vi "FormCalibra3.vi"() -> ()   [LabVIEW 2014]
uses:
  testMachine.ctl
  mainMachine.ctl
  <vilib>/Analysis/baseanly.llb/Mean (DBL).vi
  <vilib>/express/express shared/transition.llb/Dynamic To Waveform Array.vi
  <vilib>/express/express signal manip/GetorSetDDTAttributes/Set DDT Attributes/SetT0.vi
  <vilib>/express/express shared/transition.llb/Waveform Array To Dynamic.vi
  <vilib>/express/express signal manip/GetorSetDDTAttributes/Set DDT Attributes/Set DDT Properties.xnode
  <vilib>/Analysis/NI_AALBase.lvlib
panel:
  in  "buttonAcquisition":bool
  in  "editSetWaitTime":u32 caption="Tempo entre ciclos (ms)" max=999 step=1 format="%0d"
  in  "stop":bool
  out "ledSpeed":bool caption="Velocidade"
  out "error out":errorcluster
  out "ledAcquireState":bool caption="Acquire State"
  out "editTotalLowerLimit":dbl
  out "editCountLowerLimit":dbl
  out "editTotalUpperLimit":dbl
  out "editCountUpperLimit":dbl
  out "ledEnsaio 3":bool
  out "ledBrakeState":bool caption="Brake State"
  out "ledExitState":bool caption="Exit State"
  out "ledMotorState":bool caption="Motor State"
  out "ledInit2State":bool caption="Init State"
  out "ledBlockState":bool caption="Block State"
  out "ledRunningState":bool caption="Running State"
  out "ledReadyState":bool caption="Ready State"
  out "ledInitState":bool caption="Init State"
  out "mainMachine":T1
  out "testMachine":T2=enum."finish"
  in  "editSetPathToFile":path
  out "ledForce":bool caption="Célula de Carga"
  out "ledEngSpeed":bool caption="Rotação"
  out "ledTempB":bool caption="Temperatura B"
  out "ledTempA":bool caption="Temperatura A"
  out "ledTempRef":bool caption="Tempertura (Ref)"
  in  "buttonStop":bool
  in  "buttonStart":bool
  out "graphForce":dynamicdata(graph)
  in  "editOffsetForce":dbl caption="Tara" min=0.0 max=100.0 step=0.1
  in  "editSetForce":dbl caption="Fator de conversão"
  out "editForce":dbl caption="Força (Kgf)" format="%#_4f"
  out "graphSpeed":dynamicdata(graph)
  in  "editSetSpeed":dbl caption="Fator de conversão"
  out "editSpeed":dbl caption="Velocidade (km/h)" format="%#_4f"
  out "editEngineSpeed":dbl caption="Rotação (RPM)" format="%#_4f"
  in  "buttonMotor":bool
  in  "buttonBrake":bool
  in  "editSetWaitLowerTime":u32 caption="Tempo de espera (s)"
  in  "editSetWaitUpperTime":u32 caption="Tempo de espera (s)"
  in  "editSetNumberOfCycles":u32 caption="Número de ciclos" max=999 step=1 format="%0d"
  in  "editSetLowerLimit":u32 caption="Limite inferior (km/h)"
  in  "editSetUpperLimit":u32 caption="Limite superior (km/h)"
  out "editTempB":dbl caption="Temperatura B (ºC)"
  out "editTempA":dbl caption="Temperatura A (ºC)"
  in  "editSetTempRef":dbl caption="Offset referência" step=0.01 format="%#_2f"
  out "editTempRef":dbl caption="Referência (ºC)"
  out "ledMotor":bool
  out "ledBrake":bool
  out "ledEnsaio":bool
  out "labelTotalCycle":string
  out "labelCurrentCycle":string
  out "labelSystemTitle":string
  in  "editCurrCycleCtr":u32
  in  "velocidade 2":u32
  out "velocidade":u32
  # "Bancada de Frenagem - Ensaio"
  # "Sensores"
  # "Temperatura"
  # "Rotação"
  # "Célula de Carga"
  # "Configurações do ensaio"
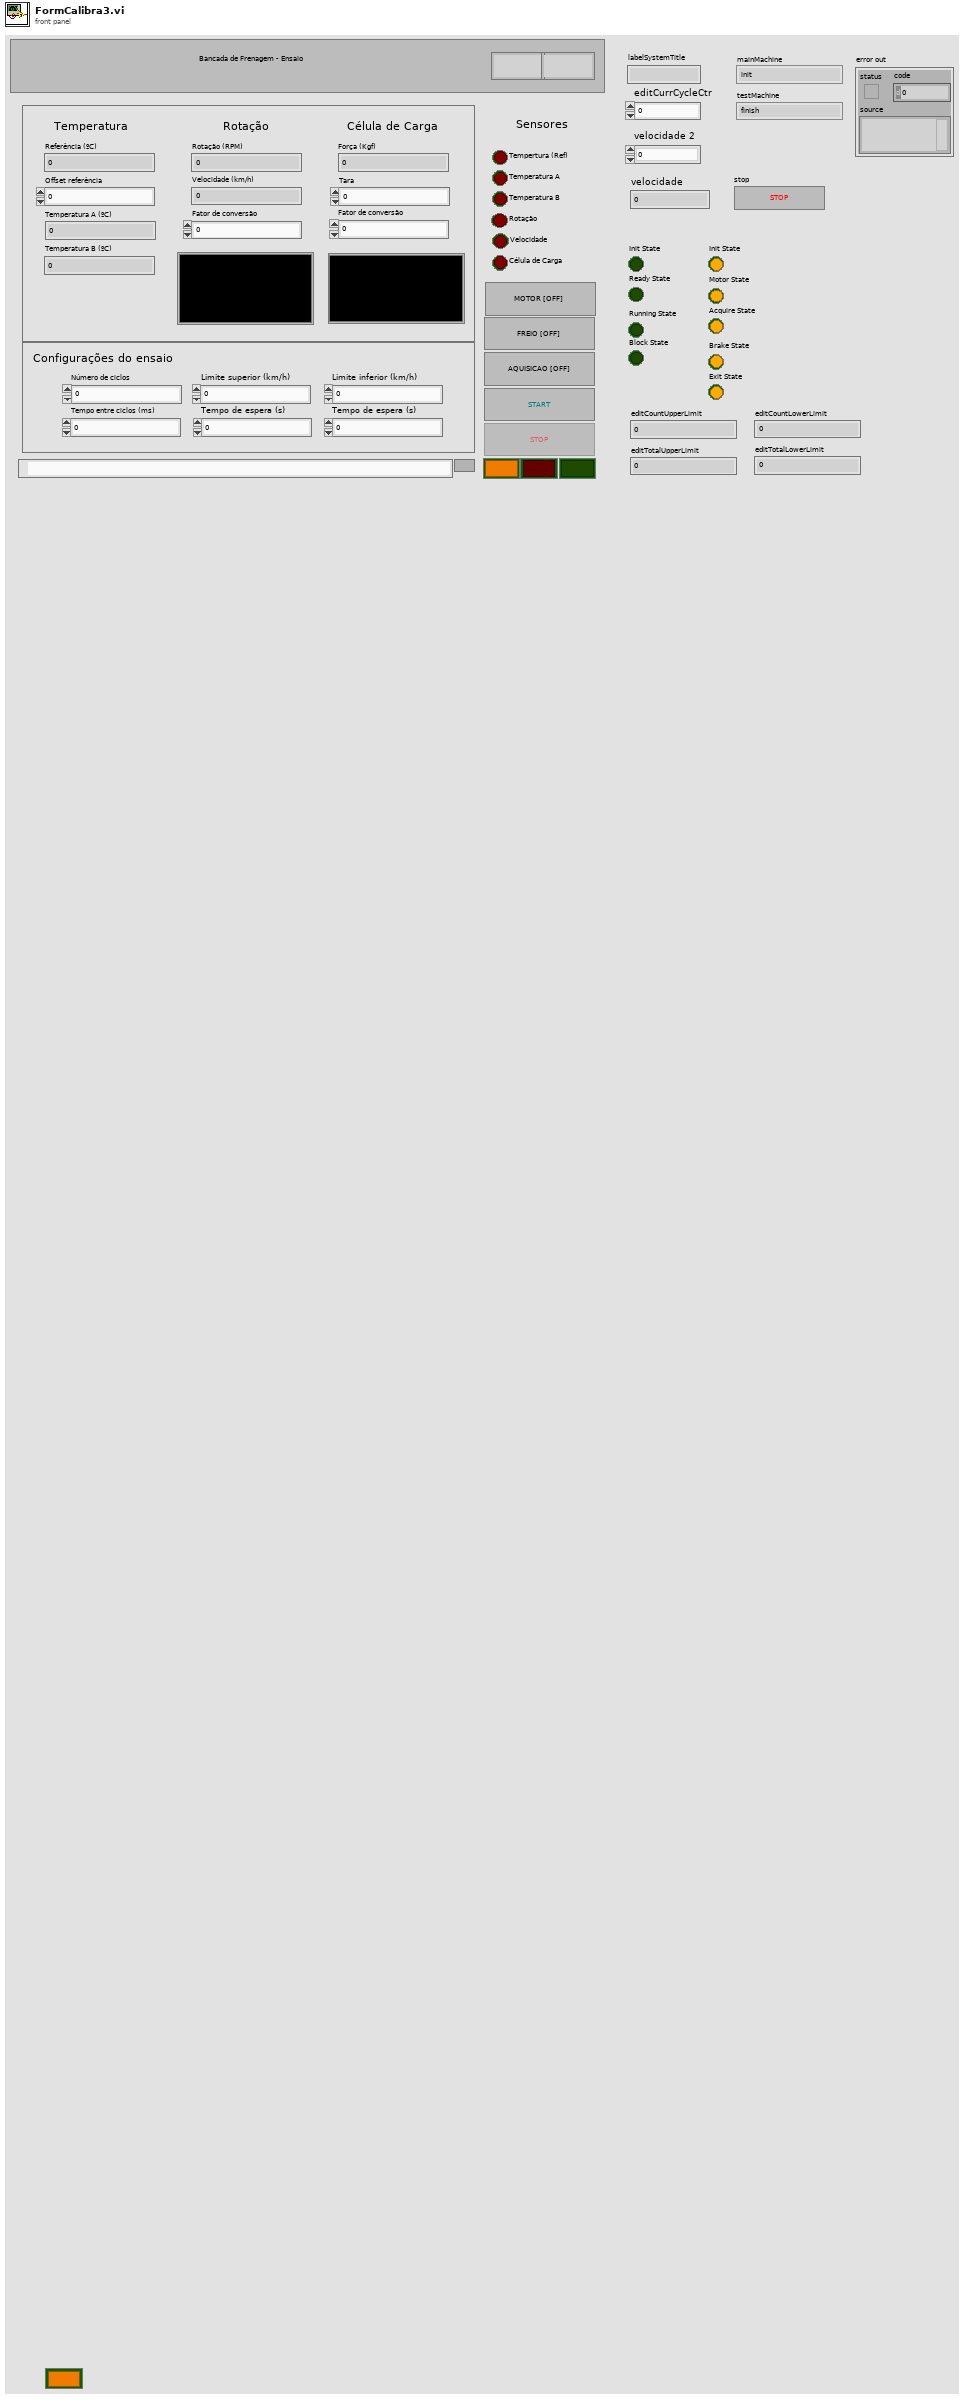
[diagram p1: front panel]
types:
  T1 = typedef "mainMachine.ctl" = enum16{"init", "ready", "running", "blocked", "finish"}
  T2 = typedef "testMachine.ctl" = enum16{"init", "motor", "motor acquire", "brake acquire", "brake", "finish", "exit"}
  T3 = enum8{"Enabled", "Disabled", "Disabled and Grayed Out"}
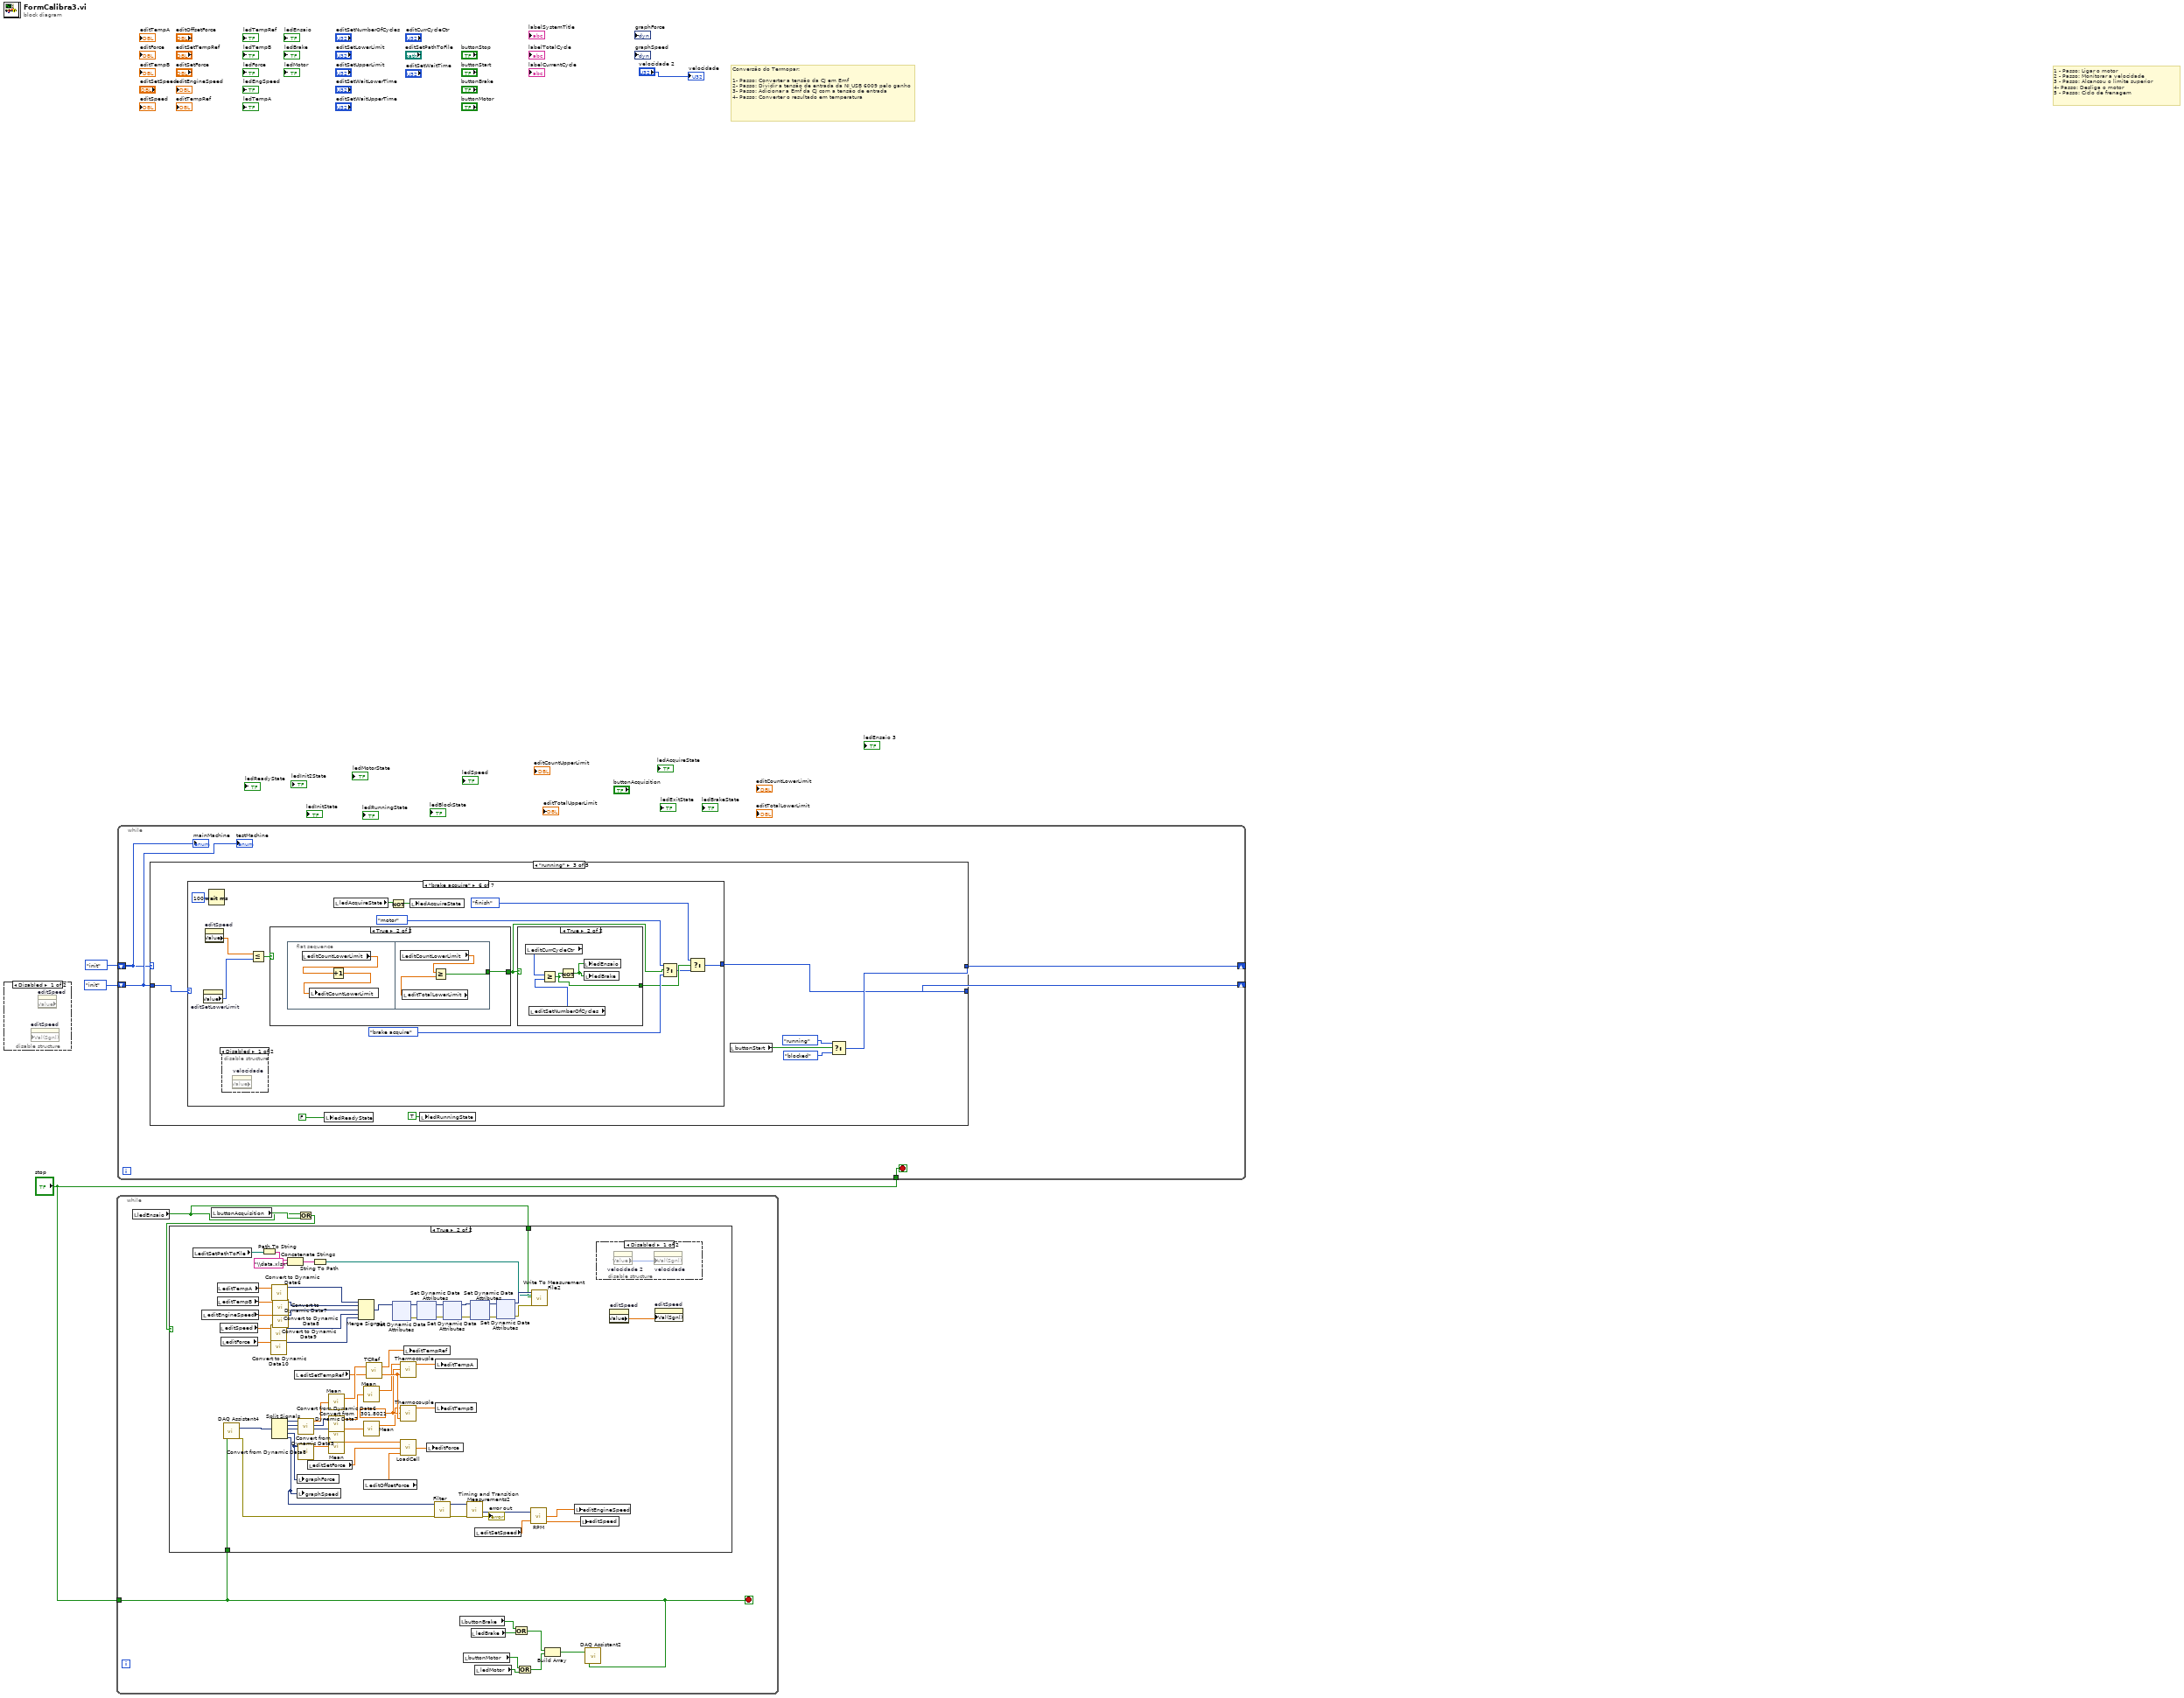
[diagram p0: block diagram]
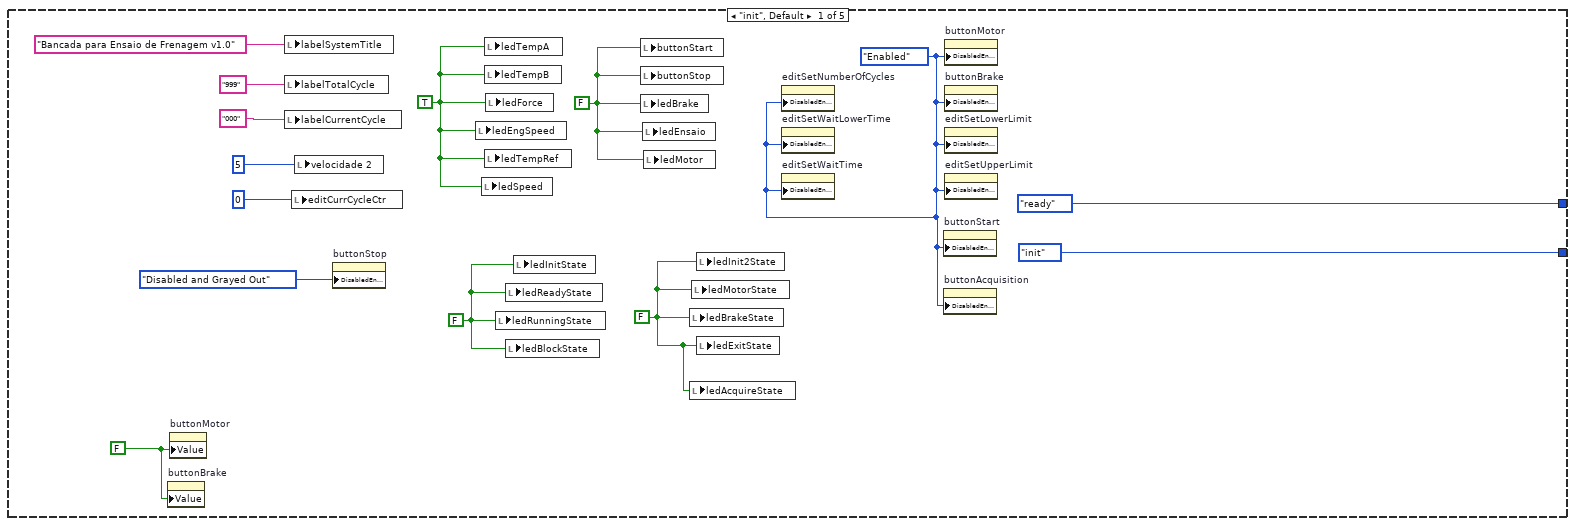
[diagram p5: hidden frame]
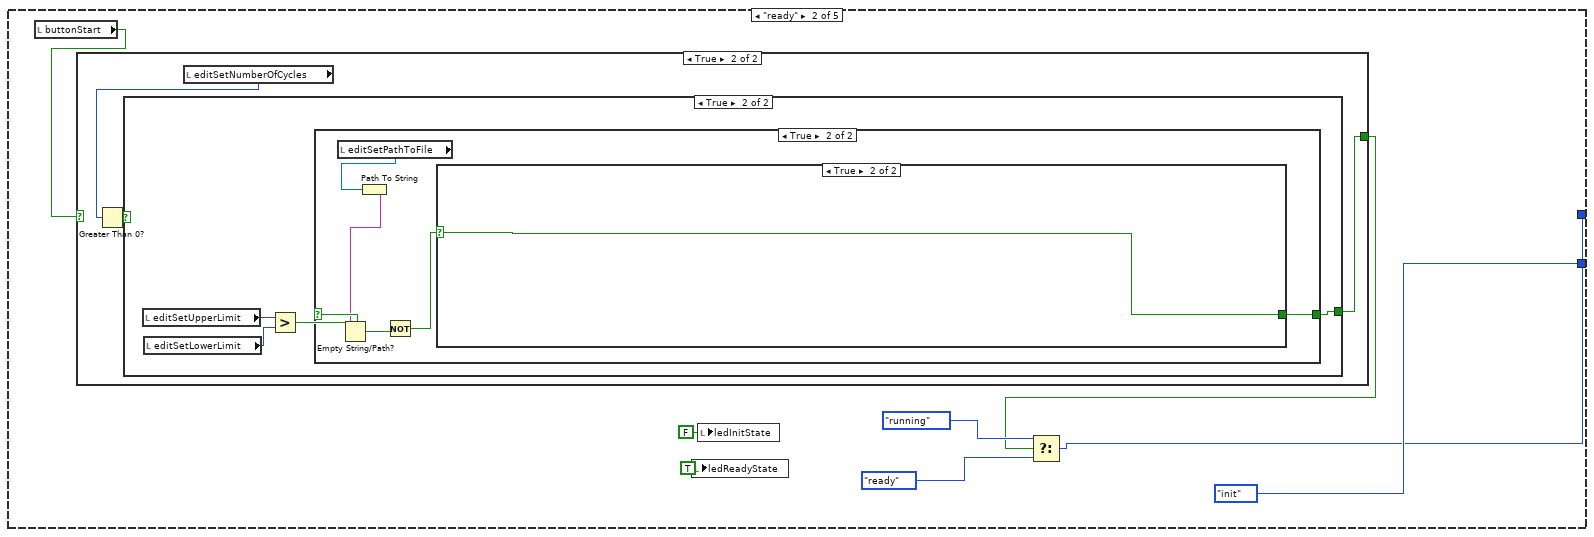
[diagram p6: hidden frame]
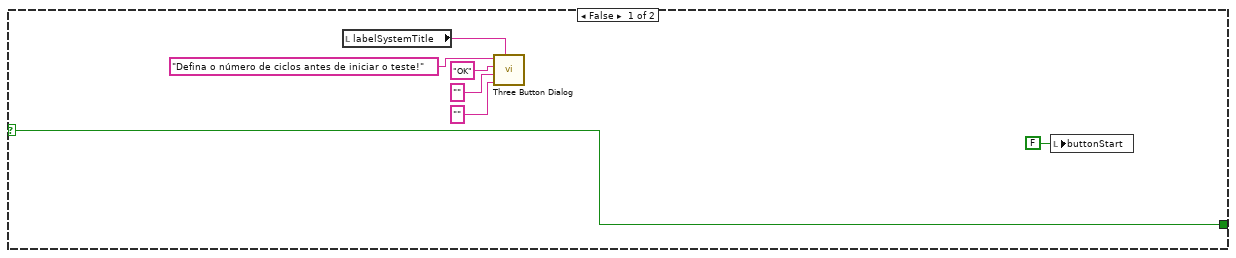
[diagram p8: hidden frame]
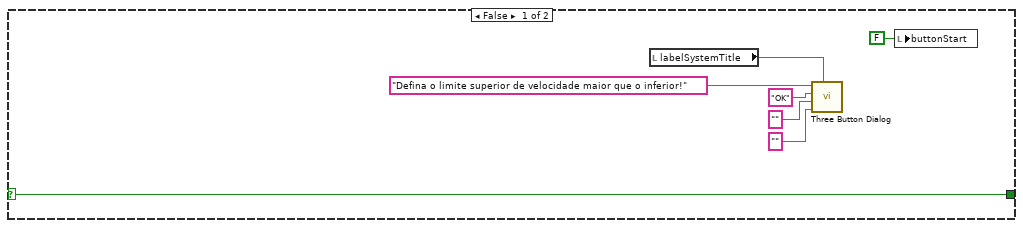
[diagram p9: hidden frame]
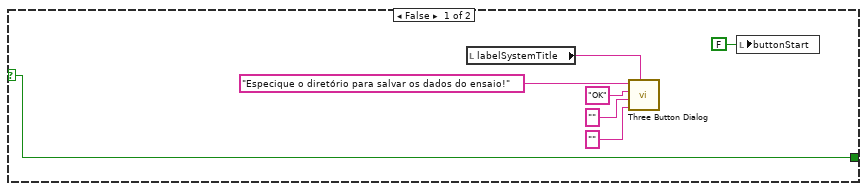
[diagram p10: hidden frame]
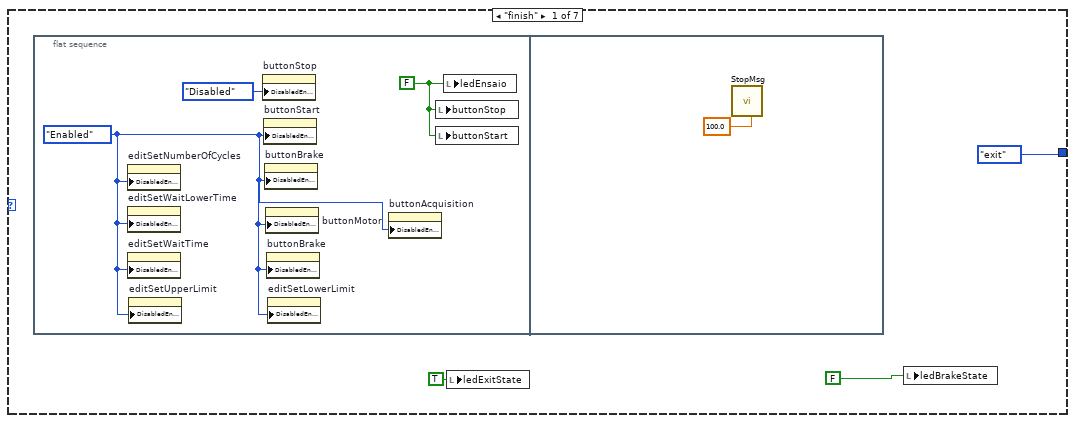
[diagram p11: hidden frame]
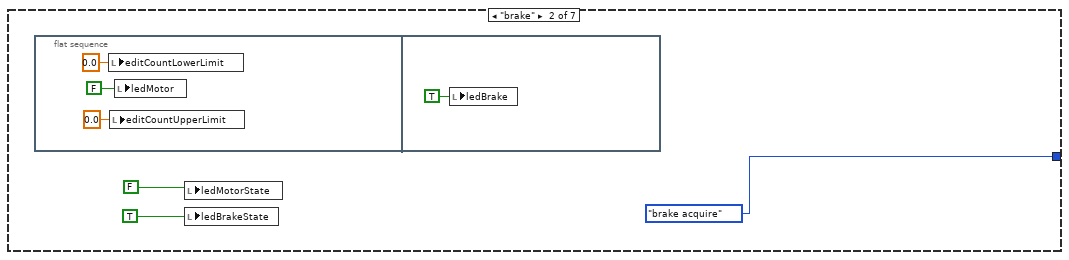
[diagram p12: hidden frame]
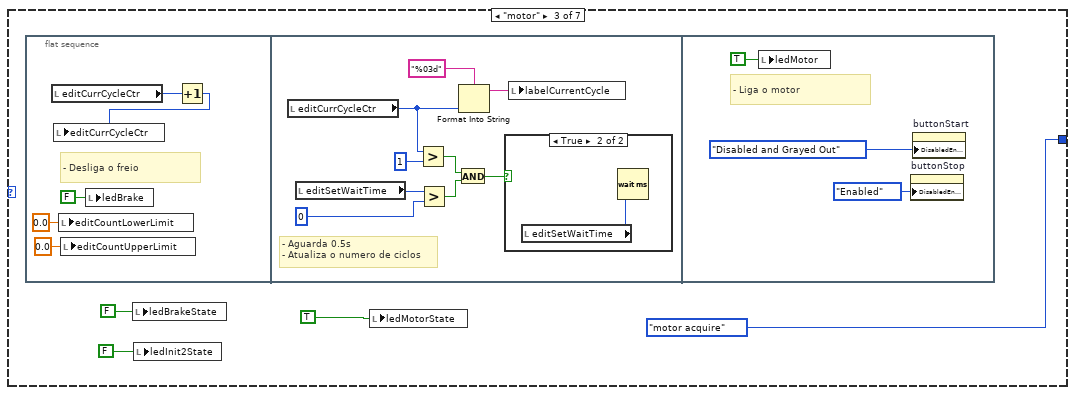
[diagram p13: hidden frame]
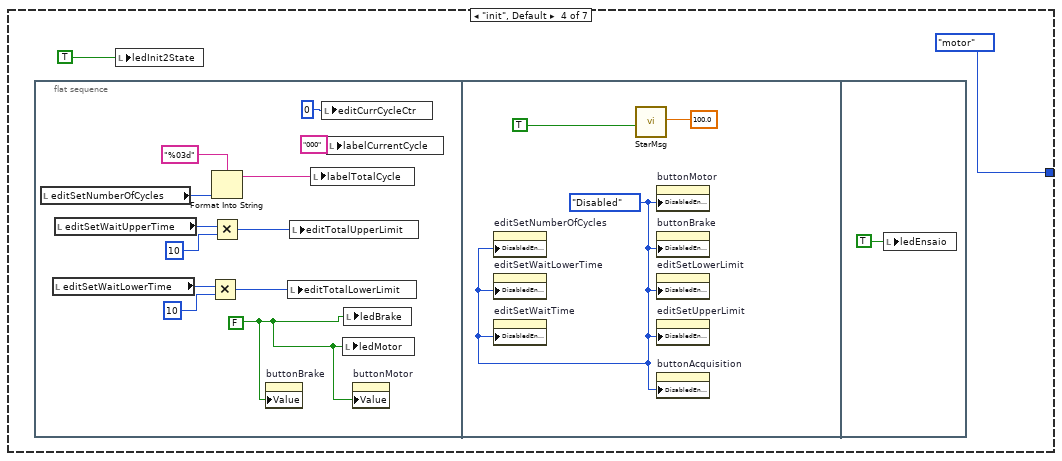
[diagram p15: hidden frame]
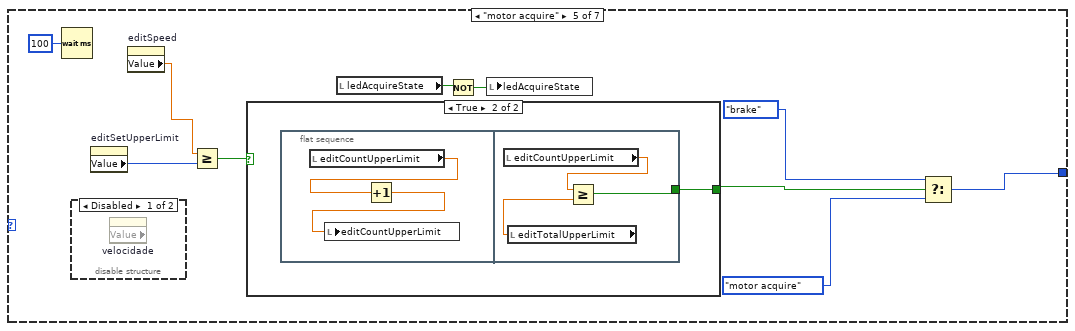
[diagram p16: hidden frame]
diagram:
  # "1 - Passo: Ligar o motor\n2 - Passo: Monitorar a velocidade\n3 - Passo: Alcancou o limite superior\n4- Passo: Desliga o motor\n5 - Passo: Ciclo de frenagem"
  # "Conversão do Termopar:\n\n1- Passo: Converter a tensão da CJ em Emf\n2- Passo: Dividir a tensão de entrada da NI USB 6009 pelo ganho\n3- Passo: Adicionar a Emf da CJ com a tensão de entrada\n4- Passo: Converter o resultado em temperatura"
  n1 = disable-structure shown="Disabled" {
    frame Disabled {
      n2 = property on="editSpeed" class="DigNum (strict)" props=["Val(Sgnl)"]() -> ()  [unwired: 3 in, 2 out]
      n3 = property on="editSpeed" class="DigNum (strict)" props=["Value"]() -> ()  [unwired: 2 in, 3 out]
    }
    frame Enabled {
    }
  }
  n4 = while {
    tunnel: "stop" -> [w8]
    stop <- w8 stop-if-true
    n5 = local read "ledEnsaio"() -> (w5:bool)
    n6 = local read "buttonAcquisition"() -> (w7:bool)
    n7 = Or(x=w5, y=w7) -> (x .or. y?=w6:bool)
    n8 = case shown="True" w6 {
      tunnel: w8 -> [_ w22]
      tunnel: w5 -> [_ w16]
      frame False {
      }
      frame True {
        w35 = 301.8021 ("factor")
        n9 = local read "editSetPathToFile"() -> (w51:path)
        n10 = local read "editEngineSpeed"() -> (w66:dbl)
        n11 = local read "editTempA"() -> (w63:dbl)
        n12 = local read "editTempB"() -> (w65:dbl)
        n13 = local read "editSpeed"() -> (w67:dbl)
        n14 = local read "editForce"() -> (w68:dbl)
        n15 = call "DAQ Assistant4"("stop (F)"=w22) -> ("data"=w24:dynamicdata, "error out"=w20:errorcluster)  [unwired: 15 in, 2 out]
        n16 = Path To String(path=w51) -> (string=w50:string)
        n17 = call "Convert to Dynamic Data9"("Double"=w67) -> ("Dynamic Data Type"=w71:dynamicdata)  [unwired: 3 in]
        n18 = call "Convert to Dynamic Data10"("Double"=w68) -> ("Dynamic Data Type"=w72:dynamicdata)  [unwired: 3 in]
        n19 = Split Signals(w24) -> (w27:dynamicdata, w31:dynamicdata, w29:dynamicdata, w40:dynamicdata, w19:dynamicdata)  [unwired: 5 in]
        n20 = call "Convert to Dynamic Data6"("Double"=w63) -> ("Dynamic Data Type"=w64:dynamicdata)  [unwired: 3 in]
        n21 = call "Convert to Dynamic Data7"("Double"=w65) -> ("Dynamic Data Type"=w69:dynamicdata)  [unwired: 3 in]
        n22 = call "Convert to Dynamic Data8"("Double"=w66) -> ("Dynamic Data Type"=w70:dynamicdata)  [unwired: 3 in]
        n23 = Concatenate Strings(w50, "\\data.xlsx" ("string")) -> (w53:string)
        n24 = local read "editSetTempRef"() -> (w26:dbl)
        n25 = local write "graphForce"(w40) -> ()
        n26 = local write "graphSpeed"(w19) -> ()
        n27 = call "Convert from Dynamic Data5"("Dynamic Data Type"=w27) -> ("Array"=w48:dbl[])  [unwired: 3 in]
        n28 = call "Convert from Dynamic Data8"("Dynamic Data Type"=w40) -> ("Array"=w32:dbl[])  [unwired: 3 in]
        n29 = local read "editSetForce"() -> (w46:dbl)
        n30 = String To Path(string=w53) -> (path=w54:path)
        n31 = call-poly <vilib>:"Mean.vi"("X"=w48) -> ("mean"=w49:dbl)  [unwired: 1 out]
        n32 = call "Convert from Dynamic Data6"("Dynamic Data Type"=w31) -> ("Array"=w28:dbl[])  [unwired: 3 in]
        n33 = call "Convert from Dynamic Data7"("Dynamic Data Type"=w29) -> ("Array"=w30:dbl[])  [unwired: 3 in]
        n34 = call-poly <vilib>:"Mean.vi"("X"=w32) -> ("mean"=w39:dbl)  [unwired: 1 out]
        n35 = Merge Signals(w64, w69, w70, w71, w72) -> (w73:dynamicdata)
        n36 = call-poly <vilib>:"Mean.vi"("X"=w28) -> ("mean"=w33:dbl)  [unwired: 1 out]
        n37 = call-poly <vilib>:"Mean.vi"("X"=w30) -> ("mean"=w34:dbl)  [unwired: 1 out]
        n38 = local read "editOffsetForce"() -> (w47:dbl)
        n39 = call "TCRef.vi"("offset"=w26, "data"=w49) -> ("emf(mV)"=w36:dbl, "temp (degC)"=w25:dbl)
        n40 = xnode ("Set Dynamic Data Attributes")("Signals In"=w73) -> ("Signals Out"=w55:dynamicdata, "error out"=w57:errorcluster)  [unwired: 4 in]
        n41 = call "Thermocouple.vi"("cj(mV)"=w36, "factor"=w35, "data"=w33) -> ("temp(degC)"=w37:dbl)  [unwired: 2 out]
        n42 = call "Thermocouple.vi"("cj(mV)"=w36, "factor"=w35, "data"=w34) -> ("temp(degC)"=w38:dbl)  [unwired: 2 out]
        n43 = call "LoadCell.vi"("tara"=w47, "factor"=w46, "data"=w39) -> ("force (Kgf)"=w43:dbl)
        n44 = local write "editTempRef"(w25) -> ()
        n45 = xnode ("Set Dynamic Data Attributes")("Signals In"=w55, "error in"=w57) -> ("Signals Out"=w56:dynamicdata, "error out"=w58:errorcluster)  [unwired: 3 in]
        n46 = local write "editForce"(w43) -> ()
        n47 = call "Filter"("error in (no error)"=w20, "Signal"=w19) -> ("error out"=w21:errorcluster, "Filtered Signal"=w18:dynamicdata)  [unwired: 8 in]
        n48 = local write "editTempA"(w37) -> ()
        n49 = local write "editTempB"(w38) -> ()
        n50 = xnode ("Set Dynamic Data Attributes")("Signals In"=w56, "error in"=w58) -> ("Signals Out"=w74:dynamicdata, "error out"=w59:errorcluster)  [unwired: 3 in]
        n51 = call "Timing and Transition Measurements2"("error in (no error)"=w21, "Signals"=w18) -> ("error out"=→"error out":errorcluster, "Frequency"=w41:dynamicdata)  [unwired: 8 in]
        n52 = xnode ("Set Dynamic Data Attributes")("Signals In"=w74, "error in"=w59) -> ("Signals Out"=w75:dynamicdata, "error out"=w60:errorcluster)  [unwired: 3 in]
        n53 = local read "editSetSpeed"() -> (w42:dbl)
        n54 = xnode ("Set Dynamic Data Attributes")("Signals In"=w75, "error in"=w60) -> ("Signals Out"=w61:dynamicdata, "error out"=w62:errorcluster)  [unwired: 3 in]
        n55 = call "RPM.vi"("data"=w41, "factor"=w42) -> ("RPM"=w44:dbl, "km/h"=w45:dbl)  [unwired: 1 out]
        n56 = call "Write To Measurement File2"("Signals"=w61, "Enable"=w16, "error in (no error)"=w62, "Filename"=w54) -> ()  [unwired: 13 in, 3 out]
        n57 = local write "editEngineSpeed"(w44) -> ()
        n58 = local write "editSpeed"(w45) -> ()
        n59 = disable-structure shown="Disabled" {
          frame Disabled {
            n60 = property on="velocidade 2" class="DigNum (strict)"() -> ("Value"=w76:u32)  [unwired: 2 in, 2 out]
            n61 = property on="velocidade" class="DigNum (strict)"("Val(Sgnl)"=w76) -> ()  [unwired: 2 in, 2 out]
          }
          frame Enabled {
          }
        }
        n62 = property on="editSpeed" class="DigNum (strict)"() -> ("Value"=w17:dbl)  [unwired: 2 in, 2 out]
        n63 = property on="editSpeed" class="DigNum (strict)"("Val(Sgnl)"=w17) -> ()  [unwired: 2 in, 2 out]
      }
    }
    n64 = local read "buttonBrake"() -> (w12:bool)
    n65 = local read "buttonMotor"() -> (w10:bool)
    n66 = local read "ledBrake"() -> (w14:bool)
    n67 = local read "ledMotor"() -> (w11:bool)
    n68 = Or(x=w12, y=w14) -> (x .or. y?=w13:bool)
    n69 = Or(x=w10, y=w11) -> (x .or. y?=w9:bool)
    n70 = Build Array(w13, w9) -> (w15:bool[])
    n71 = call "DAQ Assistant2"("data"=w15, "stop (T)"=w8) -> ()  [unwired: 16 in, 2 out]
  }
  n72 = while {
    shift-right: [w171] -> _
    shift-left: mainMachine."init" ("mainMachine") -> [w168]
    shift-right: [w170] -> _
    shift-left: testMachine."init" ("testMachine") -> [w169]
    tunnel: "stop" -> [w167]
    stop <- w167 stop-if-true
    n73 = case shown="\"running\"" w168 {
      tunnel: [mainMachine."ready" ("mainMachine") w186 w231 w334 mainMachine."finish" ("mainMachine")] -> w171
      tunnel: [testMachine."init" ("testMachine") testMachine."init" ("testMachine") w230 testMachine."init" ("testMachine") testMachine."init" ("testMachine")] -> w170
      tunnel: w169 -> [_ _ w229 _ _]
      frame "init", Default {
        w172 = T3."Enabled" ("Disabled")
        w174 = FALSE ("buttonMotor")
        w177 = FALSE
        w178 = FALSE
        w173 = TRUE
        w182 = FALSE ("motor")
        n74 = property on="buttonBrake" class="Bool (strict)"("Value"=w174) -> ()  [unwired: 2 in, 2 out]
        n75 = property on="buttonMotor" class="Bool (strict)"("Value"=w174) -> ()  [unwired: 2 in, 2 out]
        n76 = local write "labelSystemTitle"("Bancada para Ensaio de Frenagem v1.0" ("systemTitle")) -> ()
        n77 = local write "labelTotalCycle"("999" ("totalCycle")) -> ()
        n78 = local write "labelCurrentCycle"("000" ("currentCycle")) -> ()
        n79 = local write "editCurrCycleCtr"(u32 0 ("currentCycleCtr")) -> ()
        n80 = local write "velocidade 2"(u32 5 ("velocidade 2")) -> ()
        n81 = property on="buttonStop" class="Bool (strict)"("DisabledEnum"=T3."Disabled and Grayed Out" ("Disabled")) -> ()  [unwired: 2 in, 2 out]
        n82 = local write "ledEngSpeed"(w173) -> ()
        n83 = local write "ledSpeed"(w173) -> ()
        n84 = local write "ledTempA"(w173) -> ()
        n85 = local write "ledTempB"(w173) -> ()
        n86 = local write "ledTempRef"(w173) -> ()
        n87 = local write "ledForce"(w173) -> ()
        n88 = local write "ledRunningState"(w178) -> ()
        n89 = local write "ledReadyState"(w178) -> ()
        n90 = local write "ledBlockState"(w178) -> ()
        n91 = local write "ledInitState"(w178) -> ()
        n92 = local write "buttonStart"(w182) -> ()
        n93 = local write "buttonStop"(w182) -> ()
        n94 = local write "ledBrake"(w182) -> ()
        n95 = local write "ledEnsaio"(w182) -> ()
        n96 = local write "ledMotor"(w182) -> ()
        n97 = local write "ledBrakeState"(w177) -> ()
        n98 = local write "ledAcquireState"(w177) -> ()
        n99 = local write "ledMotorState"(w177) -> ()
        n100 = local write "ledInit2State"(w177) -> ()
        n101 = local write "ledExitState"(w177) -> ()
        n102 = property on="editSetNumberOfCycles" class="DigNum (strict)"("DisabledEnum"=w172) -> ()  [unwired: 2 in, 2 out]
        n103 = property on="editSetWaitLowerTime" class="DigNum (strict)"("DisabledEnum"=w172) -> ()  [unwired: 2 in, 2 out]
        n104 = property on="editSetWaitTime" class="DigNum (strict)"("DisabledEnum"=w172) -> ()  [unwired: 2 in, 2 out]
        n105 = property on="buttonStart" class="Bool (strict)"("DisabledEnum"=w172) -> ()  [unwired: 2 in, 2 out]
        n106 = property on="buttonAcquisition" class="Bool (strict)"("DisabledEnum"=w172) -> ()  [unwired: 2 in, 2 out]
        n107 = property on="buttonMotor" class="Bool (strict)"("DisabledEnum"=w172) -> ()  [unwired: 2 in, 2 out]
        n108 = property on="buttonBrake" class="Bool (strict)"("DisabledEnum"=w172) -> ()  [unwired: 2 in, 2 out]
        n109 = property on="editSetLowerLimit" class="DigNum (strict)"("DisabledEnum"=w172) -> ()  [unwired: 2 in, 2 out]
        n110 = property on="editSetUpperLimit" class="DigNum (strict)"("DisabledEnum"=w172) -> ()  [unwired: 2 in, 2 out]
      }
      frame "ready" {
        n111 = local read "buttonStart"() -> (w189:bool)
        n112 = case shown="True" w189 {
          selector: w189 -> [w194 _]
          tunnel: [w194 w195] -> w188
          frame False {
          }
          frame True {
            n113 = local read "editSetNumberOfCycles"() -> (w196:u32)
            n114 = Greater Than 0?(x=w196) -> (x > 0?=w197:bool)
            n115 = case shown="True" w197 {
              selector: w197 -> [w204 _]
              tunnel: [w204 w205] -> w195
              frame False {
                n116 = local read "labelSystemTitle"() -> (w199:string)
                n117 = call <vilib>:"Three Button Dialog.vi"("Window Title (\"\")"=w199, "Right Button Text (\"Cancel\")"="" ("Right Button Text (\"Cancel\")"), "Center Button Text (\"No\")"="" ("Center Button Text (\"No\")"), "Left Button Text (\"Yes\")"="OK" ("Left Button Text (\"Yes\")"), "message"="Defina o número de ciclos antes de iniciar o teste!") -> ()  [unwired: 6 in, 1 out]
                n118 = local write "buttonStart"(FALSE ("startButton")) -> ()
              }
              frame True {
                n119 = local read "editSetUpperLimit"() -> (w207:u32)
                n120 = local read "editSetLowerLimit"() -> (w206:u32)
                n121 = Greater?(x=w207, y=w206) -> (0:w208:bool)
                n122 = case shown="True" w208 {
                  selector: w208 -> [w215 _]
                  tunnel: [w215 w218] -> w205
                  frame False {
                    n123 = local read "labelSystemTitle"() -> (w210:string)
                    n124 = call <vilib>:"Three Button Dialog.vi"("Window Title (\"\")"=w210, "Right Button Text (\"Cancel\")"="" ("Right Button Text (\"Cancel\")"), "Center Button Text (\"No\")"="" ("Center Button Text (\"No\")"), "Left Button Text (\"Yes\")"="OK" ("Left Button Text (\"Yes\")"), "message"="Defina o limite superior de velocidade maior que o inferior!") -> ()  [unwired: 6 in, 1 out]
                    n125 = local write "buttonStart"(FALSE ("startButton")) -> ()
                  }
                  frame True {
                    n126 = local read "editSetPathToFile"() -> (w220:path)
                    n127 = Path To String(path=w220) -> (string=w219:string)
                    n128 = Empty String/Path?(string/path=w219) -> (empty?=w217:bool)
                    n129 = Not(x=w217) -> (.not. x?=w216:bool)
                    n130 = case shown="True" w216 {
                      selector: w216 -> [w227 w228]
                      tunnel: [w227 w228] -> w218
                      frame False {
                        n131 = local read "labelSystemTitle"() -> (w222:string)
                        n132 = call <vilib>:"Three Button Dialog.vi"("Window Title (\"\")"=w222, "Right Button Text (\"Cancel\")"="" ("Right Button Text (\"Cancel\")"), "Center Button Text (\"No\")"="" ("Center Button Text (\"No\")"), "Left Button Text (\"Yes\")"="OK" ("Left Button Text (\"Yes\")"), "message"="Especique o diretório para salvar os dados do ensaio!") -> ()  [unwired: 6 in, 1 out]
                        n133 = local write "buttonStart"(FALSE ("startButton")) -> ()
                      }
                      frame True {
                      }
                    }
                  }
                }
              }
            }
          }
        }
        n134 = local write "ledReadyState"(TRUE ("ledReady")) -> ()
        n135 = local write "ledInitState"(FALSE ("ledReady")) -> ()
        n136 = Select(t=mainMachine."running" ("mainMachine"), s=w188, f=mainMachine."ready" ("mainMachine")) -> (s? t:f=w186:T1)
      }
      frame "running" {
        n137 = case shown="\"brake acquire\"" w229 {
          tunnel: [testMachine."exit" ("testMachine") testMachine."brake acquire" ("testMachine") testMachine."motor acquire" ("testMachine") testMachine."motor" ("testMachine") w292 w313 testMachine."exit" ("testMachine")] -> w230
          frame "finish" {
            n138 = flat-sequence {
              frame #0 {
                w241 = FALSE ("ledReady")
                w240 = T3."Enabled" ("Disabled")
                n139 = property on="editSetNumberOfCycles" class="DigNum (strict)"("DisabledEnum"=w240) -> ()  [unwired: 2 in, 2 out]
                n140 = property on="editSetWaitLowerTime" class="DigNum (strict)"("DisabledEnum"=w240) -> ()  [unwired: 2 in, 2 out]
                n141 = property on="editSetWaitTime" class="DigNum (strict)"("DisabledEnum"=w240) -> ()  [unwired: 2 in, 2 out]
                n142 = property on="editSetUpperLimit" class="DigNum (strict)"("DisabledEnum"=w240) -> ()  [unwired: 2 in, 2 out]
                n143 = property on="buttonStop" class="Bool (strict)"("DisabledEnum"=T3."Disabled" ("Disabled")) -> ()  [unwired: 2 in, 2 out]
                n144 = property on="buttonStart" class="Bool (strict)"("DisabledEnum"=w240) -> ()  [unwired: 2 in, 2 out]
                n145 = property on="buttonBrake" class="Bool (strict)"("DisabledEnum"=w240) -> ()  [unwired: 2 in, 2 out]
                n146 = property on="buttonMotor" class="Bool (strict)"("DisabledEnum"=w240) -> ()  [unwired: 2 in, 2 out]
                n147 = property on="buttonBrake" class="Bool (strict)"("DisabledEnum"=w240) -> ()  [unwired: 2 in, 2 out]
                n148 = property on="editSetLowerLimit" class="DigNum (strict)"("DisabledEnum"=w240) -> ()  [unwired: 2 in, 2 out]
                n149 = property on="buttonAcquisition" class="Bool (strict)"("DisabledEnum"=w240) -> ()  [unwired: 2 in, 2 out]
                n150 = local write "buttonStop"(w241) -> ()
                n151 = local write "buttonStart"(w241) -> ()
                n152 = local write "ledEnsaio"(w241) -> ()
              }
              frame #1 {
                n153 = call "StopMsg.vi"("Max Value (100)"=100.0) -> ()  [unwired: 8 in, 2 out]
              }
            }
            n154 = local write "ledExitState"(TRUE ("ledReady")) -> ()
            n155 = local write "ledBrakeState"(FALSE ("ledReady")) -> ()
          }
          frame "brake" {
            n156 = flat-sequence {
              frame #0 {
                n157 = local write "editCountLowerLimit"(0.0 ("editCountUpperLimit")) -> ()
                n158 = local write "editCountUpperLimit"(0.0 ("editCountUpperLimit")) -> ()
                n159 = local write "ledMotor"(FALSE ("motor")) -> ()
              }
              frame #1 {
                n160 = local write "ledBrake"(TRUE ("freio")) -> ()
              }
            }
            n161 = local write "ledMotorState"(FALSE ("ledReady")) -> ()
            n162 = local write "ledBrakeState"(TRUE ("ledReady")) -> ()
          }
          frame "motor" {
            n163 = flat-sequence {
              frame #0 {
                # "- Desliga o freio"
                n164 = local read "editCurrCycleCtr"() -> (w258:u32)
                n165 = local write "editCountLowerLimit"(0.0 ("editCountUpperLimit")) -> ()
                n166 = local write "editCountUpperLimit"(0.0 ("editCountUpperLimit")) -> ()
                n167 = local write "ledBrake"(FALSE ("freio")) -> ()
                n168 = Increment(x=w258) -> (x+1=w257:u32)
                n169 = local write "editCurrCycleCtr"(w257) -> ()
              }
              frame #1 {
                # "- Aguarda 0.5s \n- Atualiza o numero de ciclos"
                n170 = local read "editCurrCycleCtr"() -> (w264:u32)
                n171 = local read "editSetWaitTime"() -> (w266:u32)
                n172 = Greater?(x=w264, y=u32 1) -> (0:w261:bool)
                n173 = Greater?(x=w266, y=u32 0) -> (0:w260:bool)
                n174 = And(x=w261, y=w260) -> (x .and. y?=w262:bool)
                n175 = Format Into String(format string="%03d", w264) -> (resulting string=w267:string)  [unwired: 2 in, 1 out]
                n176 = case shown="True" w262 {
                  frame False {
                  }
                  frame True {
                    n177 = local read "editSetWaitTime"() -> (w269:u32)
                    n178 = Wait (ms)(milliseconds to wait=w269) -> ()  [unwired: 1 out]
                  }
                }
                n179 = local write "labelCurrentCycle"(w267) -> ()
              }
              frame #2 {
                # "- Liga o motor"
                n180 = local write "ledMotor"(TRUE ("motor")) -> ()
                n181 = property on="buttonStop" class="Bool (strict)"("DisabledEnum"=T3."Enabled" ("Disabled")) -> ()  [unwired: 2 in, 2 out]
                n182 = property on="buttonStart" class="Bool (strict)"("DisabledEnum"=T3."Disabled and Grayed Out" ("Disabled")) -> ()  [unwired: 2 in, 2 out]
              }
            }
            n183 = local write "ledBrakeState"(FALSE ("ledReady")) -> ()
            n184 = local write "ledInit2State"(FALSE ("ledReady")) -> ()
            n185 = local write "ledMotorState"(TRUE ("ledReady")) -> ()
          }
          frame "init", Default {
            n186 = flat-sequence {
              frame #0 {
                w275 = FALSE ("ensaio")
                n187 = local read "editSetNumberOfCycles"() -> (w284:u32)
                n188 = local read "editSetWaitLowerTime"() -> (w276:u32)
                n189 = local read "editSetWaitUpperTime"() -> (w281:u32)
                n190 = Multiply(x=w276, y=u32 10) -> (x*y=w278:u32)
                n191 = Format Into String(format string="%03d", w284) -> (resulting string=w285:string)  [unwired: 2 in, 1 out]
                n192 = Multiply(x=w281, y=u32 10) -> (x*y=w279:u32)
                n193 = property on="buttonBrake" class="Bool (strict)"("Value"=w275) -> ()  [unwired: 2 in, 2 out]
                n194 = local write "editTotalLowerLimit"(w278) -> ()
                n195 = local write "editTotalUpperLimit"(w279) -> ()
                n196 = local write "labelTotalCycle"(w285) -> ()
                n197 = local write "editCurrCycleCtr"(u32 0 ("currentCycleCtr")) -> ()
                n198 = local write "labelCurrentCycle"("000" ("currentCycle")) -> ()
                n199 = local write "ledMotor"(w275) -> ()
                n200 = local write "ledBrake"(w275) -> ()
                n201 = property on="buttonMotor" class="Bool (strict)"("Value"=w275) -> ()  [unwired: 2 in, 2 out]
              }
              frame #1 {
                w287 = T3."Disabled" ("Disabled")
                n202 = property on="editSetNumberOfCycles" class="DigNum (strict)"("DisabledEnum"=w287) -> ()  [unwired: 2 in, 2 out]
                n203 = property on="editSetWaitLowerTime" class="DigNum (strict)"("DisabledEnum"=w287) -> ()  [unwired: 2 in, 2 out]
                n204 = property on="editSetWaitTime" class="DigNum (strict)"("DisabledEnum"=w287) -> ()  [unwired: 2 in, 2 out]
                n205 = call "StarMsg.vi"("Show"=TRUE, "Max Value (100)"=100.0) -> ()  [unwired: 7 in, 2 out]
                n206 = property on="buttonMotor" class="Bool (strict)"("DisabledEnum"=w287) -> ()  [unwired: 2 in, 2 out]
                n207 = property on="buttonBrake" class="Bool (strict)"("DisabledEnum"=w287) -> ()  [unwired: 2 in, 2 out]
                n208 = property on="editSetLowerLimit" class="DigNum (strict)"("DisabledEnum"=w287) -> ()  [unwired: 2 in, 2 out]
                n209 = property on="editSetUpperLimit" class="DigNum (strict)"("DisabledEnum"=w287) -> ()  [unwired: 2 in, 2 out]
                n210 = property on="buttonAcquisition" class="Bool (strict)"("DisabledEnum"=w287) -> ()  [unwired: 2 in, 2 out]
              }
              frame #2 {
                n211 = local write "ledEnsaio"(TRUE ("ensaio")) -> ()
              }
            }
            n212 = local write "ledInit2State"(TRUE ("ledReady")) -> ()
          }
          frame "motor acquire" {
            n213 = Wait (ms)(milliseconds to wait=u32 100) -> ()  [unwired: 1 out]
            n214 = disable-structure shown="Disabled" {
              frame Disabled {
                n215 = property on="velocidade" class="DigNum (strict)" props=["Value"]() -> ()  [unwired: 2 in, 3 out]
              }
              frame Enabled {
              }
            }
            n216 = property on="editSetUpperLimit" class="DigNum (strict)"() -> ("Value"=w299:u32)  [unwired: 2 in, 2 out]
            n217 = property on="editSpeed" class="DigNum (strict)"() -> ("Value"=w291:dbl)  [unwired: 2 in, 2 out]
            n218 = Greater Or Equal?(x=w291, y=w299) -> (x >= y?=w296:bool)
            n219 = case shown="True" w296 {
              selector: w296 -> [w301 _]
              tunnel: [w301 w302] -> w295
              frame False {
              }
              frame True {
                n220 = flat-sequence {
                  tunnel: [w305] -> w302
                  frame #0 {
                    n221 = local read "editCountUpperLimit"() -> (w303:dbl)
                    n222 = Increment(x=w303) -> (x+1=w304:dbl)
                    n223 = local write "editCountUpperLimit"(w304) -> ()
                  }
                  frame #1 {
                    n224 = local read "editCountUpperLimit"() -> (w307:dbl)
                    n225 = local read "editTotalUpperLimit"() -> (w306:dbl)
                    n226 = Greater Or Equal?(x=w307, y=w306) -> (x >= y?=w305:bool)
                  }
                }
              }
            }
            n227 = local read "ledAcquireState"() -> (w298:bool)
            n228 = Not(x=w298) -> (.not. x?=w297:bool)
            n229 = local write "ledAcquireState"(w297) -> ()
            n230 = Select(t=testMachine."brake" ("testMachine"), s=w295, f=testMachine."motor acquire" ("testMachine")) -> (s? t:f=w292:T2)
          }
          frame "brake acquire" {
            n231 = property on="editSetLowerLimit" class="DigNum (strict)"() -> ("Value"=w312:u32)  [unwired: 2 in, 2 out]
            n232 = property on="editSpeed" class="DigNum (strict)"() -> ("Value"=w308:dbl)  [unwired: 2 in, 2 out]
            n233 = Wait (ms)(milliseconds to wait=u32 100) -> ()  [unwired: 1 out]
            n234 = disable-structure shown="Disabled" {
              frame Disabled {
                n235 = property on="velocidade" class="DigNum (strict)" props=["Value"]() -> ()  [unwired: 2 in, 3 out]
              }
              frame Enabled {
              }
            }
            n236 = Less Or Equal?(x=w308, y=w312) -> (x <= y?=w317:bool)
            n237 = case shown="True" w317 {
              selector: w317 -> [w326 _]
              tunnel: [w326 w327] -> w315
              frame False {
              }
              frame True {
                n238 = flat-sequence {
                  tunnel: [w330] -> w327
                  frame #0 {
                    n239 = local read "editCountLowerLimit"() -> (w328:dbl)
                    n240 = Increment(x=w328) -> (x+1=w329:dbl)
                    n241 = local write "editCountLowerLimit"(w329) -> ()
                  }
                  frame #1 {
                    n242 = local read "editCountLowerLimit"() -> (w332:dbl)
                    n243 = local read "editTotalLowerLimit"() -> (w331:dbl)
                    n244 = Greater Or Equal?(x=w332, y=w331) -> (x >= y?=w330:bool)
                  }
                }
              }
            }
            n245 = local read "ledAcquireState"() -> (w319:bool)
            n246 = Not(x=w319) -> (.not. x?=w318:bool)
            n247 = local write "ledAcquireState"(w318) -> ()
            n248 = case shown="True" w315 {
              selector: w315 -> [w321 _]
              tunnel: [w321 w323] -> w311
              frame False {
              }
              frame True {
                n249 = local read "editCurrCycleCtr"() -> (w324:u32)
                n250 = local read "editSetNumberOfCycles"() -> (w325:u32)
                n251 = Greater Or Equal?(x=w324, y=w325) -> (x >= y?=w323:bool)
                n252 = Not(x=w323) -> (.not. x?=w322:bool)
                n253 = local write "ledEnsaio"(w322) -> ()
                n254 = local write "ledBrake"(w322) -> ()
              }
            }
            n255 = Select(t=testMachine."motor" ("testMachine"), s=w315, f=testMachine."brake acquire" ("testMachine")) -> (s? t:f=w310:T2)
            n256 = Select(t=testMachine."finish" ("testMachine"), s=w311, f=w310) -> (s? t:f=w313:T2)
          }
          frame "exit" {
          }
        }
        n257 = local write "ledReadyState"(FALSE ("ledReady")) -> ()
        n258 = local write "ledRunningState"(TRUE ("ledReady")) -> ()
        n259 = local read "buttonStart"() -> (w234:bool)
        n260 = Select(t=mainMachine."running" ("mainMachine"), s=w234, f=mainMachine."blocked" ("mainMachine")) -> (s? t:f=w231:T1)
      }
      frame "blocked" {
        n261 = local read "buttonStart"() -> (w338:bool)
        n262 = Select(t=mainMachine."ready" ("mainMachine"), s=w338, f=mainMachine."blocked" ("mainMachine")) -> (s? t:f=w334:T1)
        n263 = local write "ledRunningState"(FALSE ("ledReady")) -> ()
        n264 = local write "ledBlockState"(TRUE ("ledReady")) -> ()
      }
      frame "finish" {
        n265 = local write "ledBlockState"(FALSE ("ledReady")) -> ()
      }
    }
    "mainMachine" <- w168
    "testMachine" <- w169
  }
  "velocidade" <- "velocidade 2"
